vi "B-field Driver.vi"(8 "error in":errorcluster, 10 "B field(consigne)":dbl, 11 "GPIB adr in":string) -> (0 "error out":errorcluster, 2 "B field out":dbl, 3 "GPIB adr out":string)   [LabVIEW 2010]
uses:
  permanent-mode-current-value.vi
panel:
  in  "physical output channel":tag="Dev1/ao0"
  in  "ms_wait_per_halfmT":dbl
  in  "Max_Field":dbl
  in  "Coil supply":enum16{"KEPCO", "BOUHNIK"}(ring)
  in  "Emergency stop":bool
  in  "B field (goto)":dbl
  in  "stop":bool
  out "field arrived":bool
  in  "B field":dbl
  # "We're safely moving the magnetic field.\nPlease wait a little bit..."
  # "this indicator should allways have the field\nvalue of the coil\n(disregarding anything about the power supply)"
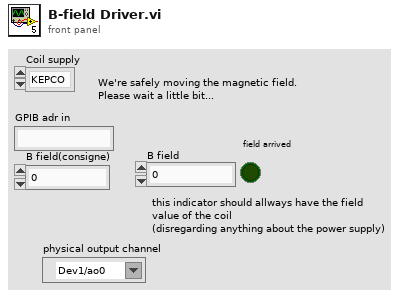
[diagram p1: front panel]
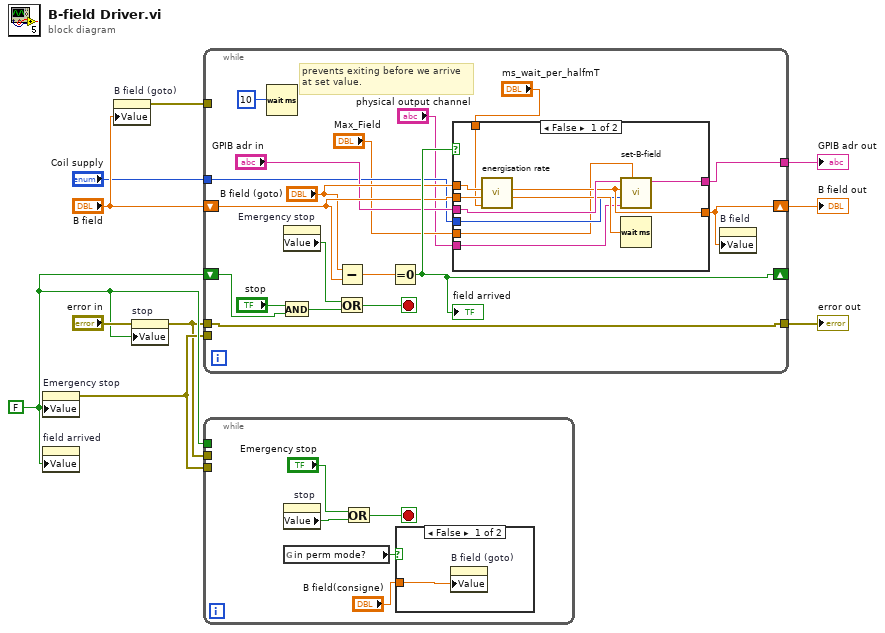
[diagram p0: block diagram]
diagram:
  w4 = FALSE ("stop")
  n1 = property on="Emergency stop" class="Bool (strict)"("Value"=w4) -> (error out=w3:errorcluster)  [unwired: 2 in, 1 out]
  n2 = property on="field arrived" class="Bool (strict)"("Value"=w4) -> ()  [unwired: 2 in, 2 out]
  n3 = property on="B field (goto)" class="DigNum (strict)"("Value"="B field") -> (error out=w5:errorcluster)  [unwired: 2 in, 1 out]
  n4 = property on="stop" class="Bool (strict)"(error in="error in", "Value"=w4) -> (error out=w2:errorcluster)  [unwired: 1 in, 1 out]
  n5 = while {
    shift-right: [w27] -> w9
    shift-left: "B field" -> [w21]
    tunnel: [w28] -> w10
    shift-right: [w22] -> _
    shift-left: w4 -> [w23]
    tunnel: w2 -> [w26]
    tunnel: [w26] -> w7
    tunnel: w5 -> [_]
    tunnel: w3 -> [_]
    tunnel: "Coil supply" -> [w14]
    stop <- w19 stop-if-true
    # "prevents exiting before we arrive\nat set value."
    n6 = Wait (ms)(milliseconds to wait=u32 10) -> ()  [unwired: 1 out]
    n7 = And(x="stop", y=w23) -> (x .and. y?=w24:bool)
    n8 = property on="Emergency stop" class="Bool (strict)"() -> ("Value"=w18:bool)  [unwired: 2 in, 2 out]
    n9 = Subtract(x="B field (goto)", y=w21) -> (x-y=w17:dbl)
    n10 = Or(x=w18, y=w24) -> (x .or. y?=w19:bool)
    n11 = Equal To 0?(x=w17) -> (x = 0?=w22:bool)
    "field arrived" <- w22
    n12 = case shown="False" w22 {
      tunnel: "GPIB adr in" -> [w38 w40]
      tunnel: [w37 w40] -> w28
      tunnel: w21 -> [w36 w39]
      tunnel: "B field (goto)" -> [w35 _]
      tunnel: [w34 w39] -> w27
      tunnel: w14 -> [w32 _]
      tunnel: "Max_Field" -> [w31 _]
      tunnel: "physical output channel" -> [w30 _]
      tunnel: "ms_wait_per_halfmT" -> [w29 _]
      frame False {
        n13 = call "energisation rate.vi"("waittime"=w29, "actual field"=w36, "B-Field (goto)"=w35) -> ("wait"=w33:dbl, "new field"=w34:dbl)  [unwired: 7 out]
        n14 = call "set-B-field.vi"("upper limit"=w31, "physical channels"=w30, "Coil supply"=w32, "Field (T)"=w34, "GPIB adr in"=w38) -> ("GPIB adr out"=w37:string)  [unwired: 6 out]
        n15 = Wait (ms)(milliseconds to wait=w33) -> ()  [unwired: 1 out]
      }
      frame True {
      }
    }
    n16 = property on="B field" class="DigNum (strict)"("Value"=w27) -> ()  [unwired: 2 in, 2 out]
  }
  "GPIB adr out" <- w10
  "B field out" <- w9
  "error out" <- w7
  n17 = while {
    tunnel: w4 -> [_]
    tunnel: w3 -> [_]
    tunnel: w2 -> [_]
    stop <- w42 stop-if-true
    n18 = property on="stop" class="Bool (strict)"() -> ("Value"=w45:bool)  [unwired: 2 in, 2 out]
    n19 = global read "permanent-mode-current-value.vi" "in perm mode?"() -> (w44:bool)
    n20 = Or(x="Emergency stop", y=w45) -> (x .or. y?=w42:bool)
    n21 = case shown="False" w44 {
      tunnel: "B field(consigne)" -> [w46 _]
      frame False {
        n22 = property on="B field (goto)" class="DigNum (strict)"("Value"=w46) -> ()  [unwired: 2 in, 2 out]
      }
      frame True {
      }
    }
  }
